vi "CheckTags.vi"(11 "UiDefinition 2":T1) -> (3 "StatusOut":refnum<vi>)   [LabVIEW 2020]
uses:
  UIReferences.ctl
  D:/LabviewDXFViewer/LabviewDXFViewer/bin/Release/LabviewDXFViewer.exe
  LabviewDXFViewer/bin/Release/LabviewDXFViewer.exe
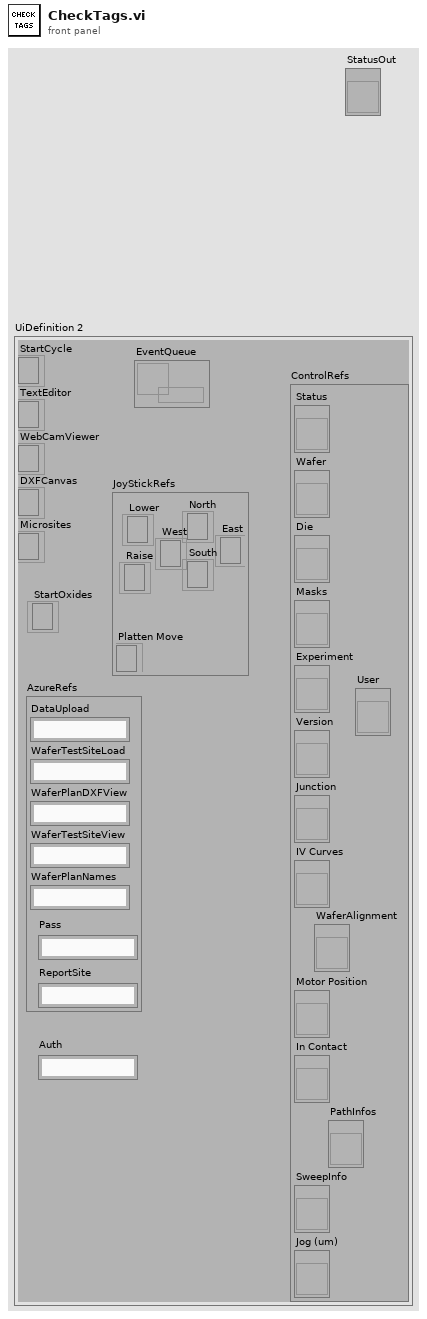
[diagram p1: front panel]
types:
  T1 = typedef "UIReferences.ctl" = cluster{"StartCycle":refnum<k24>, "TextEditor":refnum<k24>, "WebCamViewer":refnum<k24>, "DXFCanvas":refnum<k24>, "Microsites":refnum<k24>, "JoyStickRefs":cluster{"North":refnum<k24>, "Lower":refnum<k24>, "Raise":refnum<k24>, "Platten Move":refnum<k24>, "West":refnum<k24>, "East":refnum<k24>, "South":refnum<k24>}, "AzureRefs":cluster{"DataUpload":string, "WaferTestSiteLoad":string, "WaferPlanDXFView":string, "WaferTestSiteView":string, "WaferPlanNames":string, "Pass":string, "ReportSite":string}, "ControlRefs":cluster{"Status":refnum<vi>, "Wafer":refnum<vi>, "Die":refnum<vi>, "Masks":refnum<vi>, "Experiment":refnum<vi>, "Version":refnum<vi>, "Junction":refnum<vi>, "IV Curves":refnum<vi>, "Motor Position":refnum<vi>, "In Contact":refnum<vi>, "SweepInfo":refnum<vi>, "Jog (um)":refnum<vi>, "PathInfos":refnum<vi>, "User":refnum<vi>, "WaferAlignment":refnum<vi>}, "EventQueue":refnum<queue>, "StartOxides":refnum<k24>, "Auth":string}
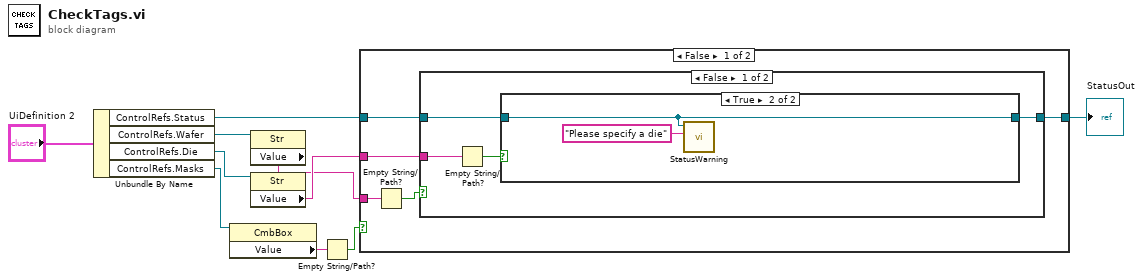
[diagram p0: block diagram]
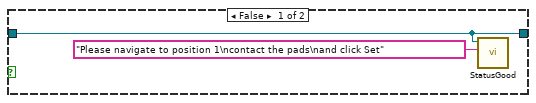
[diagram p2: hidden frame]
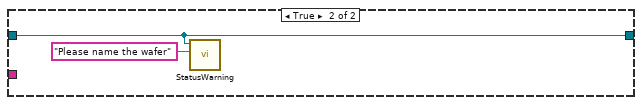
[diagram p3: hidden frame]
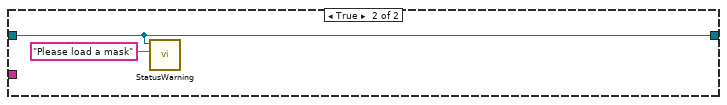
[diagram p4: hidden frame]
diagram:
  n1 = Unbundle By Name("UiDefinition 2") -> ("ControlRefs.Status"=w6:refnum<vi>, "ControlRefs.Wafer"=w5:refnum<vi>, "ControlRefs.Die"=w4:refnum<vi>, "ControlRefs.Masks"=w3:refnum<vi>)
  n2 = property class="CmbBox"(reference=w3) -> ("Value"=w8:string)  [unwired: 1 in, 2 out]
  n3 = property class="Str"(reference=w5) -> ("Value"=w1:string)  [unwired: 1 in, 2 out]
  n4 = property class="Str"(reference=w4) -> ("Value"=w2:string)  [unwired: 1 in, 2 out]
  n5 = Empty String/Path?(string/path=w8) -> (empty?=w10:bool)
  n6 = case shown="False" w10 {
    tunnel: w6 -> [w13 w26]
    tunnel: w1 -> [w15 _]
    tunnel: w2 -> [w12 _]
    tunnel: [w11 w26] -> w9
    frame False {
      n7 = Empty String/Path?(string/path=w15) -> (empty?=w14:bool)
      n8 = case shown="False" w14 {
        tunnel: w13 -> [w17 w24]
        tunnel: w12 -> [w19 _]
        tunnel: [w16 w24] -> w11
        frame False {
          n9 = Empty String/Path?(string/path=w19) -> (empty?=w18:bool)
          n10 = case shown="True" w18 {
            tunnel: w17 -> [w20 w22]
            tunnel: [w20 w22] -> w16
            frame False {
              n11 = call "StatusGood.vi"("Text.Text"="Please navigate to position 1\ncontact the pads\nand click Set", "String in"=w20) -> ()  [unwired: 10 in]
            }
            frame True {
              n12 = call "StatusWarning.vi"("Text.Text"="Please specify a die", "String in"=w22) -> ()  [unwired: 10 in]
            }
          }
        }
        frame True {
          n13 = call "StatusWarning.vi"("Text.Text"="Please name the wafer", "String in"=w24) -> ()  [unwired: 10 in]
        }
      }
    }
    frame True {
      n14 = call "StatusWarning.vi"("Text.Text"="Please load a mask", "String in"=w26) -> ()  [unwired: 10 in]
    }
  }
  "StatusOut" <- w9
